vi "그림 6-5-3 데이터로그 파일 읽기.vi"() -> ()   [LabVIEW 2010]
panel:
  out "레코드":cluster{"이름":string, "영어성적":dbl, "학번":string}[](array[cluster])
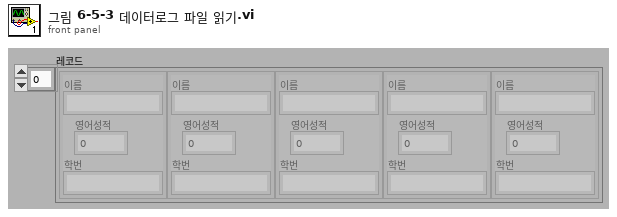
[diagram p1: front panel]
types:
  T1 = enum16{"open", "replace", "create", "open or create", "replace or create", "replace or create with confirmation"}
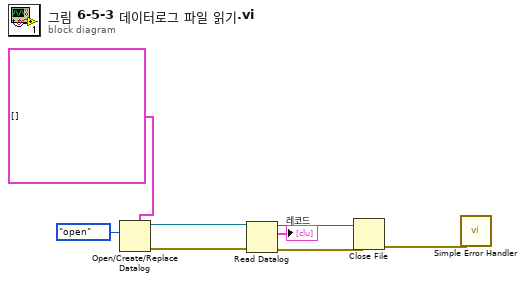
[diagram p0: block diagram]
diagram:
  n1 = Open/Create/Replace Datalog(5:cluster{"이름":string, "영어성적":dbl, "학번":string}[] [], 10:T1."open" ("동작(0:open)")) -> (0:w5:errorcluster, 3:w3:refnum<k1>)  [unwired: 4 in, 1 out]
  n2 = Read Datalog(4:w5, 7:w3) -> (0:w4:errorcluster, 2:→"레코드":cluster{"이름":string, "영어성적":dbl, "학번":string}[], 3:w2:refnum<k1>)  [unwired: 1 in]
  n3 = Close File(refnum=w2, error in=w4) -> (error out=w8:errorcluster)  [unwired: 1 out]
  n4 = call <vilib>:"Simple Error Handler.vi"("error in (no error)"=w8) -> ()  [unwired: 4 in, 5 out]
